vi "Brier_Score_Loss.vi"(8 "error in (no error)":errorcluster caption="entrée d'erreur (pas d'erreur)", 9 "y_prob":string[][](array[string]), 10 "y_true":string[][](array[string]), 11 "brier_score_loss":T1={"sample_weight"=[], "pos_label"={"dtype_pos_label"="None", "pos_label"="None"}}) -> (0 "error out":errorcluster caption="sortie d'erreur", 3 "Score":string)   [LabVIEW 2020]
doc: "Compute the Brier score.\n\nThe smaller the Brier score, the better, hence the naming with “loss”. Across all items in a set N predictions, the Brier score measures the mean squared difference between (1) the predicted probability assigned to the possible outcomes for item i, and (2) the actual outcome. Therefore, the lower the Brier score is for a set of predictions, the better the predictions are calibrated. Note that the Brier score always takes on a value between zero and one, since this is the largest possible difference between a predicted probability (which must be between zero and one) and the actual outcome (which can take on values of only 0 and 1). The Brier loss is composed of refinement loss and calibration loss. The Brier score is appropriate for binary and categorical outcomes that can be structured as true or false, but is inappropriate for ordinal variables which can take on three or more values (this is because the Brier score assumes that all possible outcomes are equivalently “distant” from one another). Which label is considered to be the positive label is controlled via the parameter pos_label, which defaults to 1.\n\n\nParameters : \n\n- y_true : array, shape (n_samples,)\nTrue targets.\n\n- y_prob : array, shape (n_samples,)\nProbabilities of the positive class.\n\n- sample_weight : array-like of shape (n_samples,), default=None\nSample weights.\n\n- pos_label : int or str, default=None\nLabel of the positive class. Defaults to the greater label unless y_true is all 0 or all -1 in which case pos_label defaults to 1.\n\nReturns : \n\n- score : float\nBrier score"
uses:
  Brier_Score_Loss.lvclass
panel:
  out "Brier_Score_Loss.lvclass":refnum<class "Brier_Score_Loss.lvclass">
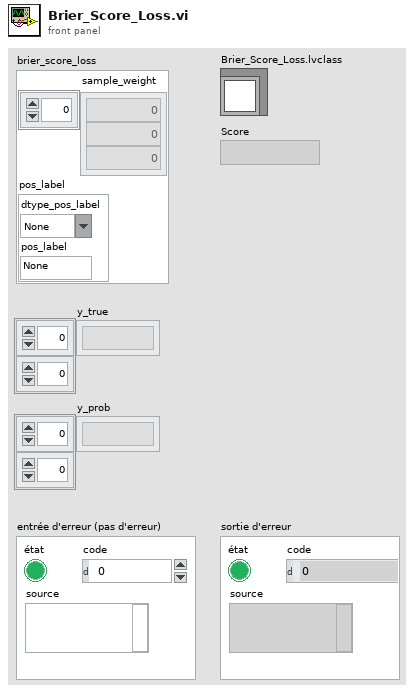
[diagram p1: front panel]
types:
  T1 = cluster{"sample_weight":dbl[], "pos_label":cluster{"dtype_pos_label":string, "pos_label":string}}
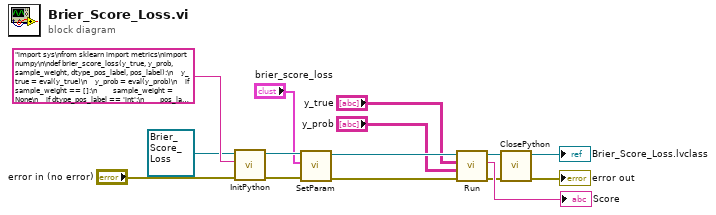
[diagram p0: block diagram]
diagram:
  n1 = call-dynamic "InitPython.vi"("error in (no error)"="error in (no error)", "Python Instruction"="import sys\nfrom sklearn import metrics\nimport numpy\n\ndef brier_score_loss(y_true, y_prob, sample_weight, dtype_pos_label, pos_label):\n    y_true = eval(y_true)\n    y_prob = eval(y_prob)\n    if sample_weight == []:\n        sample_weight = None\n    if dtype_pos_label == 'int':\n        pos_label = eval(pos_label)\n    elif dtype_pos_label == 'None':\n        pos_label = None\n    try:\n        brier_score_loss = metrics.brier_score_loss(y_true, y_prob, sample_weight, pos_label)\n        brier_score_loss = brier_score_loss.tolist()\n        return str(brier_score_loss)\n    except:\n        erreur = sys.exc_info()\n        typerr = u\"%s\" % (erreur[0])\n        typerr = typerr[typerr.find(\"'\")+1:typerr.rfind(\"'\")]\n        msgerr = u\"%s\" % (erreur[1])\n        message = str('/!\\\\ {0} : {1}'. format(typerr,msgerr))\n        return message", "Scikit-learn en entrée"=refnum<class "Brier_Score_Loss.lvclass"> refnum ("Brier_Score_Loss.lvclass")) -> ("error out"=w10:errorcluster, "Scikit-learn en sortie"=w11:refnum<class "Brier_Score_Loss.lvclass">)  [unwired: 7 in]
  n2 = call-dynamic "SetParam.vi"("error in (no error)"=w10, "brier_score_loss"="brier_score_loss", "Brier_Score_Loss.lvclass"=w11) -> ("error out"=w7:errorcluster, "Brier_Score_Loss.lvclass"=w8:refnum<class "Brier_Score_Loss.lvclass">)  [unwired: 7 in]
  n3 = call-dynamic "Run.vi"("error in (no error)"=w7, "y_prob"="y_prob", "y_true"="y_true", "Brier_Score_Loss.lvclass"=w8) -> ("error out"=w4:errorcluster, "Score"=→"Score":string, "Brier_Score_Loss.lvclass"=w6:refnum<class "Brier_Score_Loss.lvclass">)  [unwired: 5 in]
  n4 = call-dynamic "ClosePython.vi"("error in (no error)"=w4, "Scikit-learn en entrée"=w6) -> ("error out"=→"error out":errorcluster, "Scikit-learn en sortie"=→"Brier_Score_Loss.lvclass":refnum<class "Brier_Score_Loss.lvclass">)  [unwired: 8 in]
